vi "DAQmx(AI).TestLauncher.vi"() -> ()   [LabVIEW 2013, in "DAQmx(AI).lvclass"]
doc: "JKI State Machine Objects (SMO) 1.0.0.5\nJKI - JKI\nCopyright (c) 2016, JKI"
uses:
  DAQmx(AI).lvclass
  Typedefs/Scaling(MapRange)--Cluster.ctl
  Typedefs/InputConfiguration--Cluster.ctl
  Typedefs/Units -- Enum.ctl
  <vilib>/JKI/JKI SMO/SMO/Typedefs/SMOState --Enum.ctl
  Set Scaling (MapRange).vi
  <vilib>/JKI/JKI SMO/SMO/SMO.lvclass
panel:
  out "Waveform Chart":dbl(graph) caption="Waveform Graph"
  in  "Physical Channel":tag="SMO-Sim/ai0"
  out "Device Name":tag="SMO-Sim"
  out "Simulated":bool
  out "Device found":bool
  out "error out":errorcluster
  in  "Stop":bool
  # "Analog Input DAQmx Test Launcher"
  # "For instructions on how to use the JKI State Machine Objects, examples and video tutorials, visit:\nhttp://jki.net/state-machine-objects/\n\nJKI State Machine Objects™\nhttp://jki.net/state-machine-objects/\nCopyright (C) 2005-2016, JKI <info@jki.net>\nALL RIGHTS RESERVED"
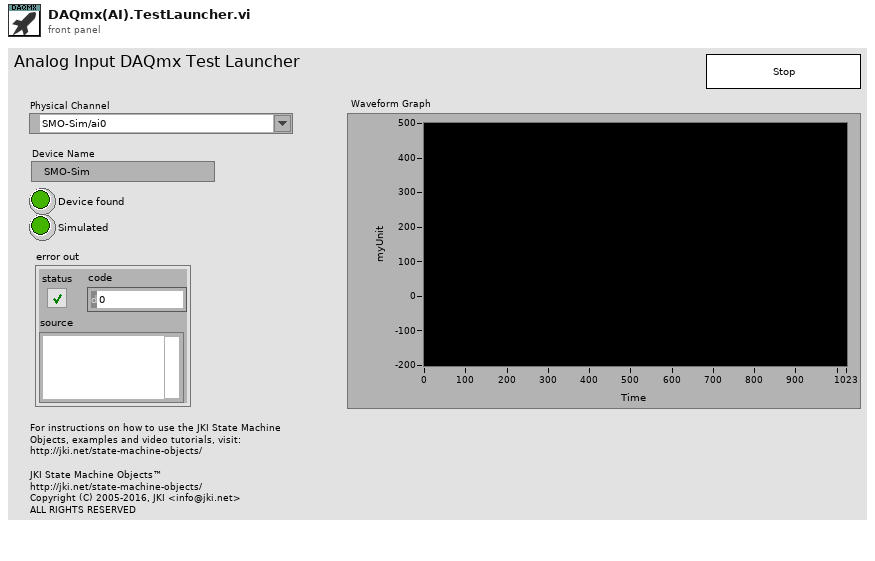
[diagram p1: front panel]
types:
  T1 = typedef "DAQmx(AI).lvclass/InputConfiguration--Cluster.ctl" = cluster{"input terminal":i32, "minimum value":dbl, "maximum value":dbl, "units":T2}
  T2 = typedef "DAQmx(AI).lvclass/Units -- Enum.ctl" = enum16{"Volts", "Amps", "Deg F", "Deg C", "Deg R", "Kelvins", "Strain", "Ohms", "Hz", "Seconds", "Meters", "Inches", "Degrees", "Radians", "Ticks", "g", "m/s^2", "m/s", "in/s", "Pascals", "Newtons", "Pounds", "kgf", "psi", "bar", "Nm", "oz-in", "lb-in", "lb-ft", "Volts/Volt", "mVolts/Volt", "From TEDS"}
  T3 = typedef "DAQmx(AI).lvclass/Scaling(MapRange)--Cluster.ctl" = cluster{"Minimum":dbl, "Maximum":dbl}
  T4 = typedef "DAQmx(AI).lvclass/PublicEvents--Cluster.ctl" = cluster{"Value Changed":refnum<user-event>, "Task Configuration":refnum<user-event>, "Scaling":refnum<user-event>}
  T5 = typedef "SMO.lvclass/Public Events.ctl" = cluster{"Error":refnum<user-event>, "State":refnum<user-event>}
  T6 = typedef "SMO.lvclass/SMOState --Enum.ctl" = enum16{"unknown", "Created", "Started", "Stopped"}
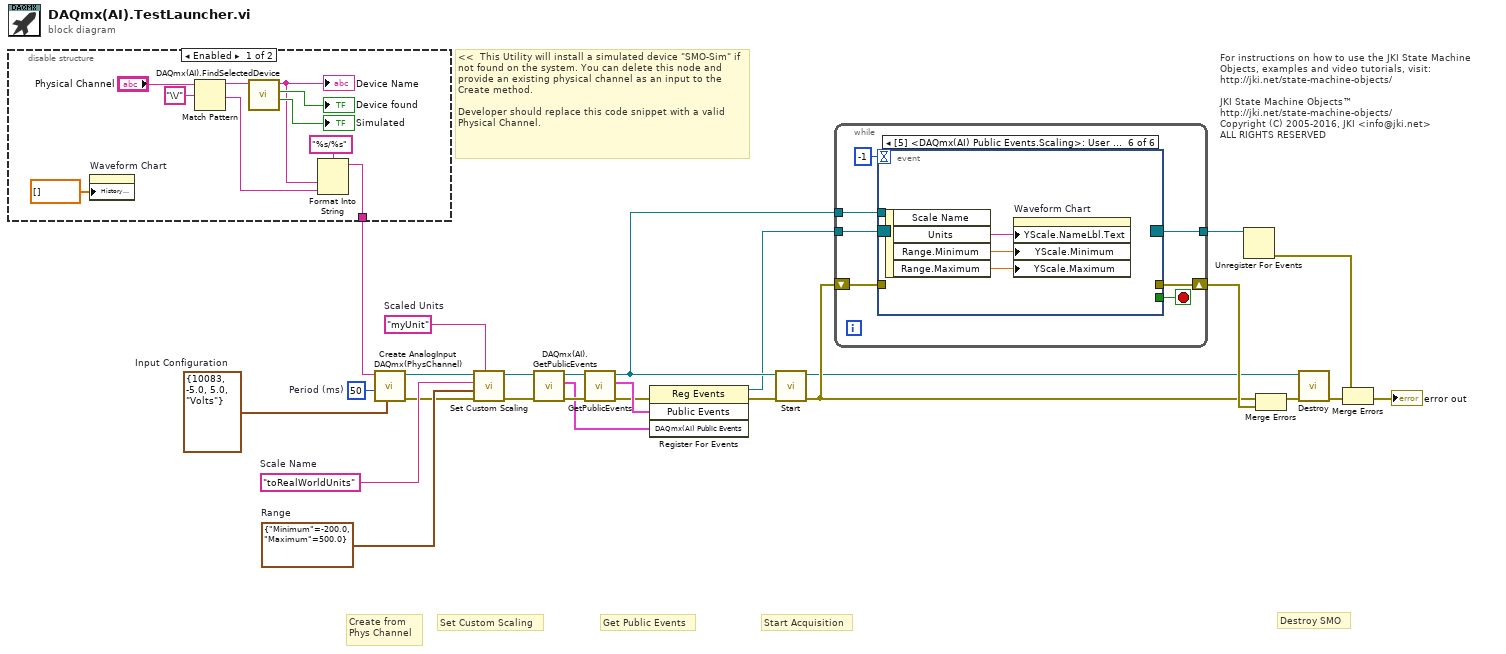
[diagram p0: block diagram]
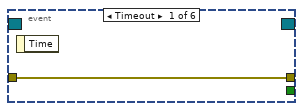
[diagram p3: hidden frame]
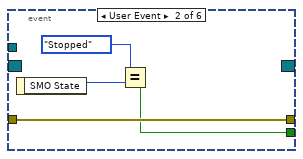
[diagram p4: hidden frame]
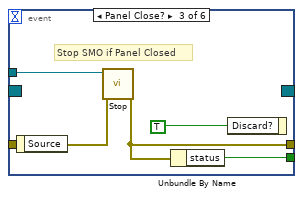
[diagram p5: hidden frame]
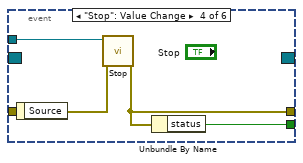
[diagram p6: hidden frame]
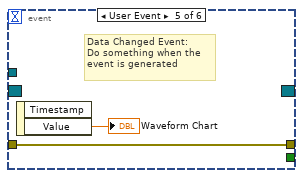
[diagram p7: hidden frame]
diagram:
  w1 = T1 {"input terminal"=10083, "minimum value"=-5.0, "maximum value"=5.0, "units"=enum."Volts"}  # Input Configuration
  w2 = "myUnit"  # Scaled Units
  w5 = T3 {"Minimum"=-200.0, "Maximum"=500.0}  # Range
  w6 = "toRealWorldUnits"  # Scale Name
  w10 = i64 50  # Period (ms)
  # "Create from\nPhys Channel"
  # "Set Custom Scaling"
  # "<<  This Utility will install a simulated device \"SMO-Sim\" if not found on the system. You can delete this node and provide an existing physical channel as an input to the Create method.\n\nDeveloper should replace this code snippet with a valid Physical Channel."
  # "For instructions on how to use the JKI State Machine Objects, examples and video tutorials, visit:\nhttp://jki.net/state-machine-objects/\n\nJKI State Machine Objects™\nhttp://jki.net/state-machine-objects/\nCopyright (C) 2005-2016, JKI <info@jki.net>\nALL RIGHTS RESERVED"
  # "Get Public Events"
  # "Start Acquisition"
  # "Destroy SMO"
  n1 = disable-structure shown="Enabled" {
    disable-tunnel: [w28 _] -> w9
    frame Enabled {
      n2 = property on="Waveform Chart" class="WFChart (strict)"("History Data"=dbl[] []) -> ()  [unwired: 2 in, 2 out]
      n3 = Match Pattern(string="Physical Channel", regular expression="\\/") -> (before substring=w32:string, after substring=w30:string)  [unwired: 1 in, 2 out]
      n4 = call "DAQmx(AI).FindSelectedDevice.vi"("Device Name"=w32) -> ("Simulated"=→"Simulated":bool, "Device found"=→"Device found":bool, "ActiveDev"=w31:tag)  [unwired: 7 in, 1 out]
      "Device Name" <- w31
      n5 = Format Into String(format string="%s/%s", w31, w30) -> (resulting string=w28:string)  [unwired: 2 in, 1 out]
    }
    frame Disabled {
    }
  }
  n6 = call "Create AnalogInput DAQmx(PhysChannel).vi"("Input Configuration"=w1, "Period (ms)"=w10, "DAQmx Physical Channel"=w9) -> ("error out"=w4:errorcluster, "Subsystem out"=w8:refnum<class "DAQmx(AI).lvclass">)  [unwired: 6 in, 1 out]
  n7 = call-poly "Set Custom Scaling.vi"("Scaled Units"=w2, "error in (no error)"=w4, "Map Range"=w5, "Scale Name"=w6, "DAQmx(AI) in"=w8) -> ("error out"=w3:errorcluster, "DAQmx(AI) out"=w7:refnum<class "DAQmx(AI).lvclass">)  [unwired: 5 in]
  n8 = call "DAQmx(AI).GetPublicEvents.vi"("error in (no error)"=w3, "Subsystem"=w7) -> ("error out"=w13:errorcluster, "DAQmx(AI) Public Events"=w11:T4, "Subsystem out"=w12:refnum<class "DAQmx(AI).lvclass">)  [unwired: 7 in]
  n9 = call <vilib>:"GetPublicEvents.vi"("error in (no error)"=w13, "SMO"=w12) -> ("error out"=w15:errorcluster, "Public Events"=w16:T5, "SMO out"=w18:refnum<class "DAQmx(AI).lvclass">)  [unwired: 7 in]
  n10 = register-events(error in=w15, w16, w11) -> (reference out=w14:refnum<event-registration>, error out=w17:errorcluster)  [unwired: 1 in]
  n11 = call <vilib>:"Start.vi"("error in (no error)"=w17, "SMO"=w18) -> ("error out"=w21:errorcluster, "SMO out"=w19:refnum<class "DAQmx(AI).lvclass">)  [unwired: 8 in]
  n12 = while {
    shift-right: [w42] -> w25
    shift-left: w21 -> [w41]
    tunnel: w14 -> [w40]
    tunnel: [w39] -> w26
    tunnel: w18 -> [w38]
    stop <- w43 stop-if-true
    n13 = event shown="[5] <DAQmx(AI) Public Events.Scaling>: User Event" {
      selector: w40 -> [_ _ _ _ _ _]
      dyn-events: [_ _ _ _ _ _] -> w39
      timeout: -1 -> [_ _ _ _ _ _]
      tunnel: [_ w45 w49 w54 _ _] -> w43
      tunnel: w38 -> [_ _ w53 w57 _ _]
      tunnel: [w44 w48 w50 w55 w59 _] -> w42
      tunnel: w41 -> [w44 w48 w52 w56 w59 _]
      event Timeout {
        n14 = event-data() -> ()  [unwired: 1 in, 1 out]
      }
      event User Event {
        n15 = event-data() -> ("SMO State"=w47:T6)  [unwired: 1 in]
        n16 = Equal?(x=SMOState_--Enum."Stopped", y=w47) -> (x = y?=w45:bool)
      }
      event Panel Close? {
        # "Stop SMO if Panel Closed"
        n17 = event-data() -> ()  [unwired: 1 in, 1 out]
        n18 = call <vilib>:"Stop.vi"("error in (no error)"=w52, "SMO"=w53) -> ("error out"=w50:errorcluster)  [unwired: 8 in, 1 out]
        n19 = Unbundle By Name(w50) -> ("status"=w49:bool)
        n20 = event-data("Discard?"=TRUE ("OK")) -> ()  [unwired: 1 in, 1 out]
      }
      event "Stop": Value Change {
        n21 = event-data() -> ()  [unwired: 1 in, 1 out]
        n22 = call <vilib>:"Stop.vi"("error in (no error)"=w56, "SMO"=w57) -> ("error out"=w55:errorcluster)  [unwired: 8 in, 1 out]
        n23 = Unbundle By Name(w55) -> ("status"=w54:bool)
      }
      event User Event {
        # "Data Changed Event:\nDo something when the\nevent is generated"
        n24 = event-data() -> ("Value"=→"Waveform Chart":dbl)  [unwired: 1 in, 1 out]
      }
      event User Event {
        n25 = event-data() -> ("Units"=w62:string, "Range.Minimum"=w61:dbl, "Range.Maximum"=w60:dbl)  [unwired: 1 in, 1 out]
        n26 = property on="Waveform Chart" class="WFChart (strict)"("YScale.NameLbl.Text"=w62, "YScale.Minimum"=w61, "YScale.Maximum"=w60) -> ()  [unwired: 2 in, 2 out]
      }
    }
  }
  n27 = Unregister For Events(event registration refnum=w26) -> (error out=w24:errorcluster)  [unwired: 1 in]
  n28 = Merge Errors(w21, w25) -> (w20:errorcluster)
  n29 = call <vilib>:"Destroy.vi"("error in (no error)"=w20, "SMO"=w19) -> ("error out"=w22:errorcluster)  [unwired: 9 in]
  n30 = Merge Errors(w24, w22) -> (→"error out":errorcluster)
